vi "Save Load Settings.vi"(0 "VISA resource name":refnum<visa-resource-name>, 5 "Save/Load (T: Load)":bool, 7 "Load? (0:Default Settings)":T1(ring), 9 "Save as? (0: SAV0)":enum16{"SAV0", "SAV1", "SAV2", "SAV3", "SAV4"}(ring), 11 "error in (no error)":errorcluster, 12 "Power-on Setup (F: OFF)":bool) -> (4 "VISA resource name out":refnum<visa-resource-name>, 15 "error out":errorcluster)   [LabVIEW 2017, in "Keithley 3390.lvlib"]
doc: "Saves/loads the current instrument settings to/from memory."
uses:
  Keithley 3390.lvlib
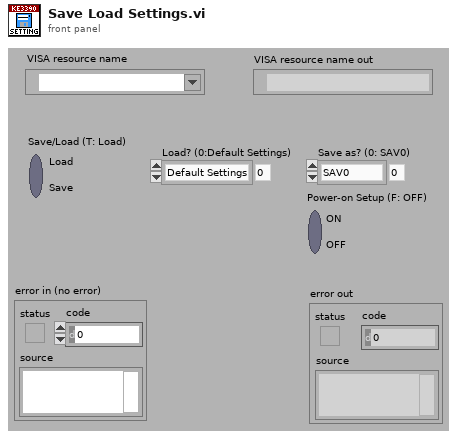
[diagram p1: front panel]
types:
  T1 = enum16{"Default Settings", "SAV0", "SAV1", "SAV2", "SAV3", "SAV4"}
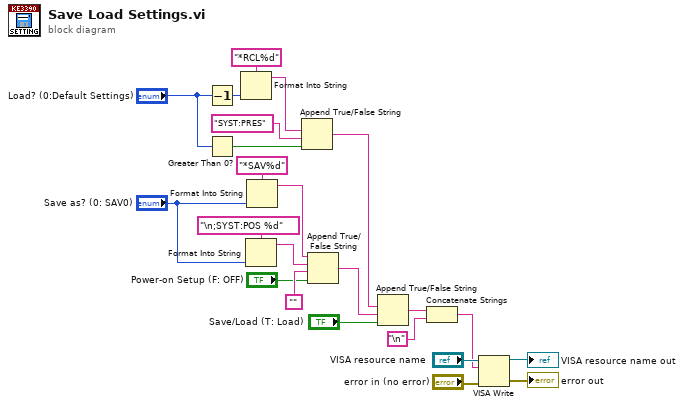
[diagram p0: block diagram]
diagram:
  n1 = Decrement(x="Load? (0:Default Settings)") -> (x-1=w20:T1)
  n2 = Greater Than 0?(x="Load? (0:Default Settings)") -> (x > 0?=w19:bool)
  n3 = Format Into String(format string="*RCL%d", w20) -> (resulting string=w18:string)  [unwired: 2 in, 1 out]
  n4 = Format Into String(format string="\n;SYST:POS %d", "Save as? (0: SAV0)") -> (resulting string=w10:string)  [unwired: 2 in, 1 out]
  n5 = Format Into String(format string="*SAV%d", "Save as? (0: SAV0)") -> (resulting string=w14:string)  [unwired: 2 in, 1 out]
  n6 = Append True/False String(1:w19, 2:"SYST:PRES" ("format string"), 3:w18) -> (0:w15:string)  [unwired: 1 in]
  n7 = Append True/False String(1:"Power-on Setup (F: OFF)", 2:"", 3:w10, 4:w14) -> (0:w8:string)
  n8 = Append True/False String(1:"Save/Load (T: Load)", 2:w8, 3:w15) -> (0:w3:string)  [unwired: 1 in]
  n9 = Concatenate Strings(w3, "\n") -> (w1:string)
  n10 = VISA Write(VISA resource name="VISA resource name", write buffer=w1, error in (no error)="error in (no error)") -> (VISA resource name out=→"VISA resource name out":refnum<visa-resource-name>, error out=→"error out":errorcluster)  [unwired: 1 out]
